vi "str to security policy.vi"(11 "trimmed string":string) -> (3 "security policy":T1)   [LabVIEW 2014, in "OPCUA XML(dev).lvlib"]
uses:
  OPCUA XML(dev).lvlib
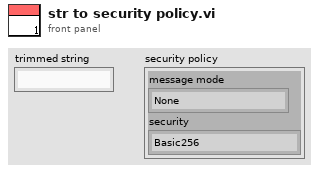
[diagram p1: front panel]
types:
  T1 = cluster{"message mode":enum16{"None", "Sign", "Sign and Encrypt"}, "security":enum16{"Basic256", "Basic128Rsa15"}}
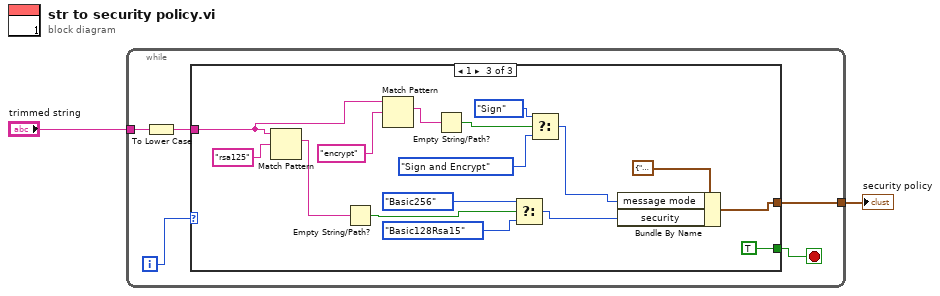
[diagram p0: block diagram]
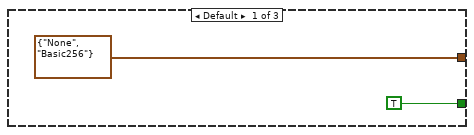
[diagram p2: hidden frame]
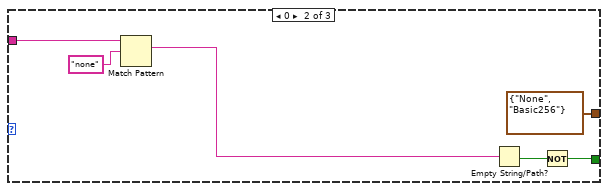
[diagram p3: hidden frame]
diagram:
  n1 = while {
    tunnel: "trimmed string" -> [w7]
    tunnel: [w4] -> w1
    i -> [w5]
    stop <- w3 stop-if-true
    n2 = To Lower Case(string=w7) -> (all lower case string=w6:string)
    n3 = case shown="1" w5 {
      tunnel: w6 -> [_ w15 w26]
      tunnel: [TRUE w13 TRUE] -> w3
      tunnel: [T1 {"message mode"=enum."None", "security"=enum."Basic256"} ("security policy") T1 {"message mode"=enum."None", "security"=enum."Basic256"} ("security policy") w17] -> w4
      frame Default {
      }
      frame 0 {
        n4 = Match Pattern(string=w15, regular expression="none") -> (match substring=w11:string)  [unwired: 1 in, 3 out]
        n5 = Empty String/Path?(string/path=w11) -> (empty?=w12:bool)
        n6 = Not(x=w12) -> (.not. x?=w13:bool)
      }
      frame 1 {
        n7 = Match Pattern(string=w26, regular expression="rsa125") -> (match substring=w30:string)  [unwired: 1 in, 3 out]
        n8 = Empty String/Path?(string/path=w30) -> (empty?=w27:bool)
        n9 = Match Pattern(string=w26, regular expression="encrypt") -> (match substring=w24:string)  [unwired: 1 in, 3 out]
        n10 = Empty String/Path?(string/path=w24) -> (empty?=w21:bool)
        n11 = Select(t=enum16{"Basic256", "Basic128Rsa15"}."Basic256" ("security"), s=w27, f=enum16{"Basic256", "Basic128Rsa15"}."Basic128Rsa15" ("security")) -> (s? t:f=w18:enum16{"Basic256", "Basic128Rsa15"})
        n12 = Select(t=enum16{"None", "Sign", "Sign and Encrypt"}."Sign" ("message mode"), s=w21, f=enum16{"None", "Sign", "Sign and Encrypt"}."Sign and Encrypt" ("message mode")) -> (s? t:f=w19:enum16{"None", "Sign", "Sign and Encrypt"})
        n13 = Bundle By Name(cluster=T1 {"message mode"=enum."None", "security"=enum."Basic256"} ("security policy"), "message mode"=w19, "security"=w18) -> (w17:T1)
      }
    }
  }
  "security policy" <- w1
